vi "Set Isolated Crop Mode Ex.vi"(4 "cropbottom":i32, 5 "cropleft":i32, 6 "hbin":i32, 7 "vbin":i32, 8 "error in (no error)":errorcluster, 9 "cropwidth":i32, 10 "cropheight":i32, 11 "active":i32) -> (0 "error out":errorcluster, 3 "function return":u32)   [LabVIEW 2014, in "atmcd32d.lvlib"]
doc: "unsigned int WINAPI SetIsolatedCropModeEx(int active, int cropheight, int cropwidth, int vbin, int hbin, int cropleft, int cropbottom);"
uses:
  atmcd32d.lvlib
  atmcd32d.dll
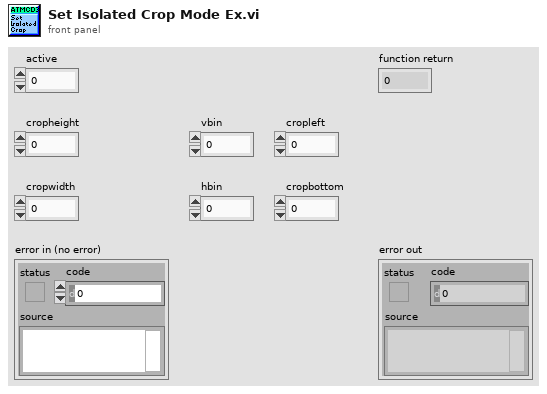
[diagram p1: front panel]
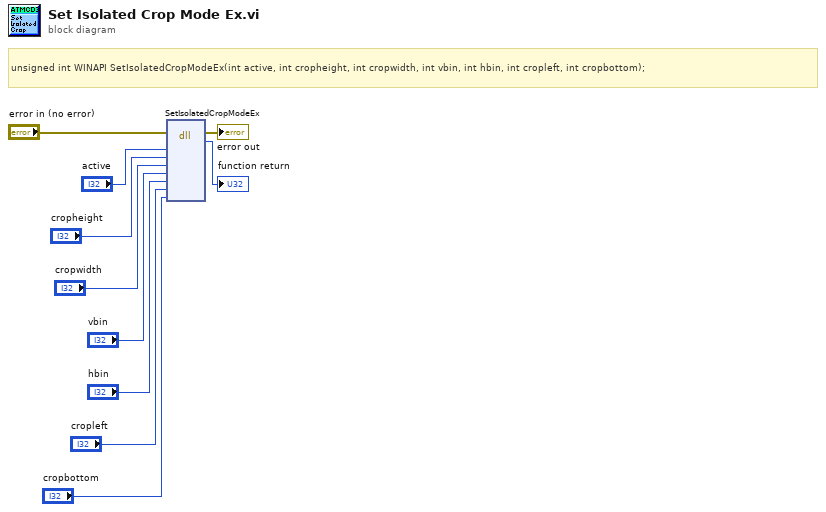
[diagram p0: block diagram]
diagram:
  # "unsigned int WINAPI SetIsolatedCropModeEx(int active, int cropheight, int cropwidth, int vbin, int hbin, int cropleft, int cropbottom);"
  n1 = dll-call lib="C:/Users/Bakir/Documents/Lambda2-Testing/lib/Andorlib/atmcd32d.*" fn="SetIsolatedCropModeEx"(error in="error in (no error)", "active"="active", "cropheight"="cropheight", "cropwidth"="cropwidth", "vbin"="vbin", "hbin"="hbin", "cropleft"="cropleft", "cropbottom"="cropbottom") -> (error out=→"error out":errorcluster, →"function return":u32)  [unwired: 9 in, 1 out]
